vi "FileIO-Create Backup.vi"(6 "Append date":bool, 8 "error in (no error)":errorcluster, 9 "Subfolder":string, 10 "Delete tag":bool, 11 "Path":path) -> (0 "error out":errorcluster, 1 "backup created?":bool, 2 "Backup Path":path, 3 "Path (thru)":path)   [LabVIEW 2020]
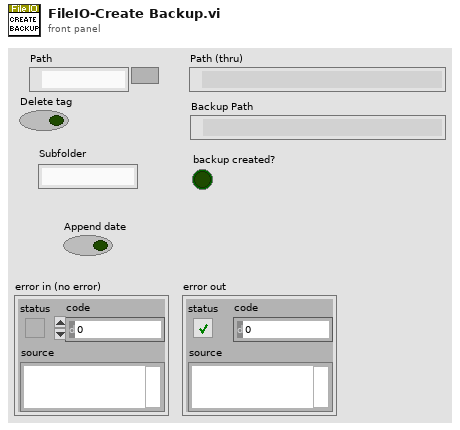
[diagram p1: front panel]
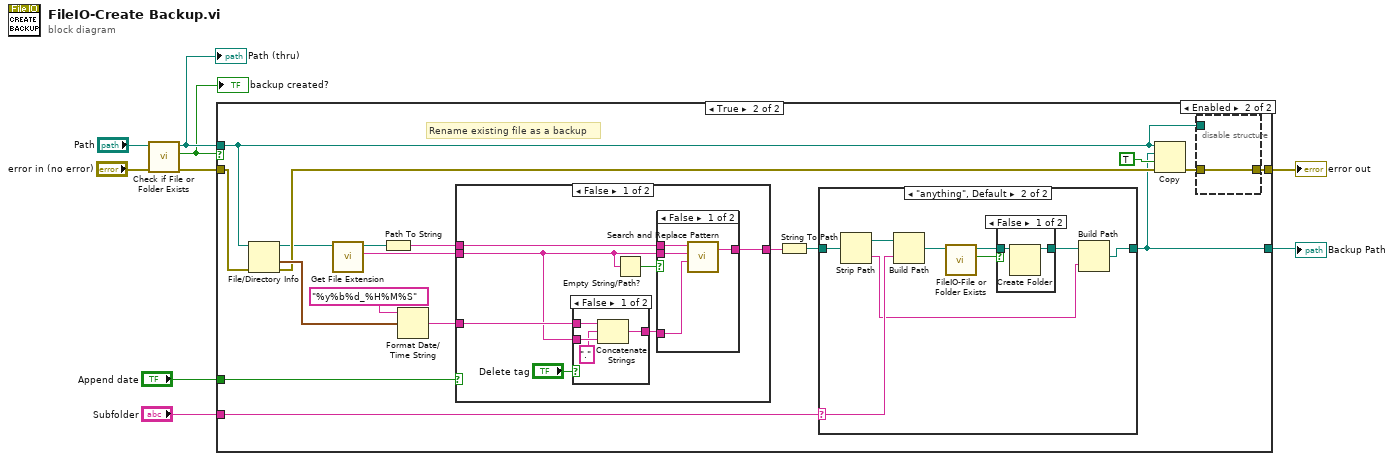
[diagram p0: block diagram]
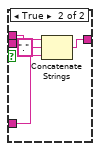
[diagram p5: hidden frame]
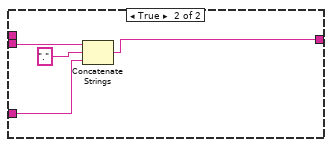
[diagram p7: hidden frame]
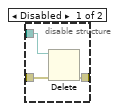
[diagram p8: hidden frame]
diagram:
  n1 = call <vilib>:"Check if File or Folder Exists.vi"("error in (no error)"="error in (no error)", "path"="Path") -> ("error out"=w6:errorcluster, "file or folder exists?"=w5:bool, "dup path"=w9:path)  [unwired: 7 in]
  "Path (thru)" <- w9
  "backup created?" <- w5
  n2 = case shown="True" w5 {
    tunnel: w9 -> [_ w21]
    tunnel: w6 -> [w10 w19]
    tunnel: [w10 w22] -> w7
    tunnel: [_ w11] -> w4
    tunnel: "Append date" -> [_ w14]
    tunnel: "Subfolder" -> [_ w12]
    frame False {
    }
    frame True {
      # "Rename existing file as a backup"
      n3 = File/Directory Info(path=w21, error in=w19) -> (path out=w17:path, last mod=w23:timestamp, error out=w18:errorcluster)  [unwired: 4 out]
      n4 = call <vilib>:"Get File Extension.vi"("file"=w17) -> ("lowercase file extension"=w15:string, "dup file"=w16:path)  [unwired: 6 in, 3 out]
      n5 = Path To String(path=w16) -> (string=w28:string)
      n6 = Format Date/Time String(time format string (%c)="%y%b%d_%H%M%S", seconds (now)=w23) -> (date/time string=w27:string)  [unwired: 1 in]
      n7 = case shown="False" w14 {
        tunnel: w28 -> [w48 w65]
        tunnel: w27 -> [w47 w64]
        tunnel: [w45 w62] -> w26
        tunnel: w15 -> [w42 _]
        frame False {
          n8 = case shown="False" "Delete tag" {
            tunnel: w47 -> [w60 w61]
            tunnel: [w59 w61] -> w46
            tunnel: w42 -> [w58 _]
            frame False {
              n9 = Concatenate Strings(w60, "." ("string"), w58) -> (w59:string)
            }
            frame True {
            }
          }
          n10 = Empty String/Path?(string/path=w42) -> (empty?=w43:bool)
          n11 = case shown="False" w43 {
            tunnel: w48 -> [w52 w56]
            tunnel: w46 -> [w51 w54]
            tunnel: [w50 w55] -> w45
            tunnel: w42 -> [w49 _]
            frame False {
              n12 = call <vilib>:"Search and Replace Pattern.vi"("string"=w52, "regular expression (\"\")"=w49, "replace string (\"\")"=w51) -> ("result string"=w50:string)  [unwired: 2 in, 1 out]
            }
            frame True {
              n13 = Concatenate Strings(w56, "." ("string"), w54) -> (w55:string)
            }
          }
        }
        frame True {
          n14 = Concatenate Strings(w65, "." ("string"), w64) -> (w62:string)
        }
      }
      n15 = String To Path(string=w26) -> (path=w13:path)
      n16 = case shown="\"anything\", Default" w12 {
        selector: w12 -> [_ w36]
        tunnel: w13 -> [w29 w38]
        tunnel: [w29 w34] -> w11
        frame "" {
        }
        frame "anything", Default {
          n17 = Strip Path(path=w38) -> (stripped path=w37:path, name=w35:string)
          n18 = Build Path(base path=w37, name or relative path=w36) -> (appended path=w32:path)
          n19 = call "FileIO-File or Folder Exists.vi"("path"=w32) -> ("Directory?"=w31:bool, "dup path"=w30:path)  [unwired: 7 in, 2 out]
          n20 = case shown="False" w31 {
            tunnel: [w40 w41] -> w33
            tunnel: w30 -> [w39 w41]
            frame False {
              n21 = Create Folder(path (use dialog)=w39) -> (created path=w40:path)  [unwired: 2 in, 2 out]
            }
            frame True {
            }
          }
          n22 = Build Path(base path=w33, name or relative path=w35) -> (appended path=w34:path)
        }
      }
      n23 = Copy(8:w18, 9:TRUE ("overwrite (F)"), 10:w11, 11:w21) -> (0:w25:errorcluster)  [unwired: 1 in, 2 out]
      n24 = disable-structure shown="Enabled" {
        disable-tunnel: w25 -> [w68 w69]
        disable-tunnel: [w67 w69] -> w22
        disable-tunnel: w21 -> [w66 _]
        frame Disabled {
          n25 = Delete(path (use dialog)=w66, error in=w68) -> (error out=w67:errorcluster)  [unwired: 3 in, 2 out]
        }
        frame Enabled {
        }
      }
    }
  }
  "error out" <- w7
  "Backup Path" <- w4
